vi "DetectQRCodesARGB.vi"(8 "error in (no error)":errorcluster, 10 "ARGB Image":refnum<data-value>, 11 "QRCodeDetector in":refnum<class "QRDetector.lvclass">) -> (0 "error out":errorcluster, 2 "Detections":T1[](array[typedef]), 3 "QRCodeDetector (Duplicate)":refnum<class "QRDetector.lvclass">)   [LabVIEW 2020, in "g_ar_toolkit.feature_detection.lvlib" / "QRDetector.lvclass"]
uses:
  QRDetector.lvclass
  Detection.ctl
  Detection Region.ctl
  g_ar_toolkit.common/Image Point (Float).ctl
  QRDetector.lvclass/QRDetector.ctl
  g_ar_toolkit.common/Module Path.vi
  <vilib>/Utility/error.llb/Error Cluster From Error Code.vi
  947807d6-cf22-42cc-b024-3c0d53b5d2ed.vi
  g_ar_toolkit.common/g_ar_toolkit.common.lvlib
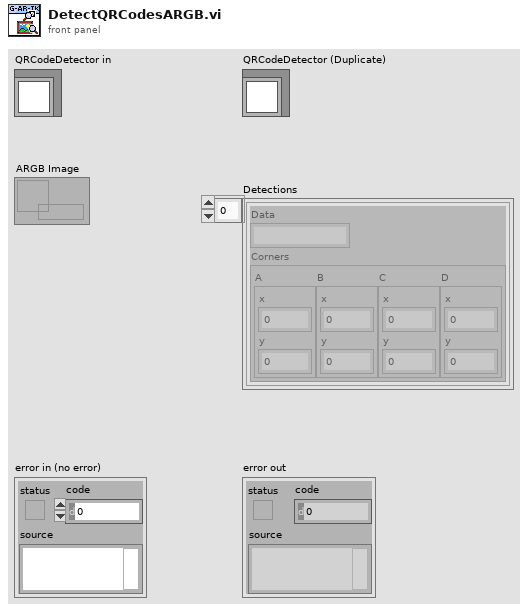
[diagram p1: front panel]
types:
  T1 = typedef "g_ar_toolkit.feature_detection.lvlib/QRDetector.lvclass/Detection.ctl" = cluster{"Data":string, "Corners":T2}
  T2 = typedef "g_ar_toolkit.feature_detection.lvlib/QRDetector.lvclass/Detection Region.ctl" = cluster{"A":T3, "B":T3, "C":T3, "D":T3}
  T3 = typedef "g_ar_toolkit.common.lvlib/Image Point (Float).ctl" = cluster{"x":dbl, "y":dbl}
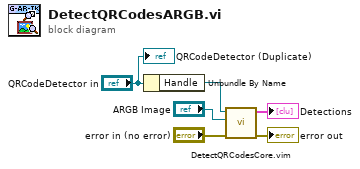
[diagram p0: block diagram]
diagram:
  n1 = Unbundle By Name("QRCodeDetector in") -> ("Handle"=w1:refnum<data-value>)
  n2 = call "DetectQRCodesCore.vim"("error in (no error)"="error in (no error)", "Greyscale Image"="ARGB Image", "Handle"=w1) -> ("error out"=→"error out":errorcluster, "Detections"=→"Detections":T1[])  [unwired: 7 in]
  "QRCodeDetector (Duplicate)" <- "QRCodeDetector in"
